vi "Start test 1.vi"(8 "error in (no error)":errorcluster, 11 "Test_ExampleClassA in":refnum<class "Test_ExampleClassA.lvclass">) -> (0 "error out":errorcluster, 3 "Test_ExampleClassA out":refnum<class "Test_ExampleClassA.lvclass">)   [LabVIEW 2012, in "Test_ExampleClassA.lvclass"]
doc: "Starts test 1 (i.e. the second default test). Sends an update command together with a complete set of settings to test whether an acknowledge command is returned."
uses:
  Test_ExampleClassA.lvclass
  Test settings cluster.ctl
  ExampleClassA/Settings cluster.ctl
  MurmexTest/MurmexTest.lvclass
  ExampleClassA/ExampleClassA.lvclass
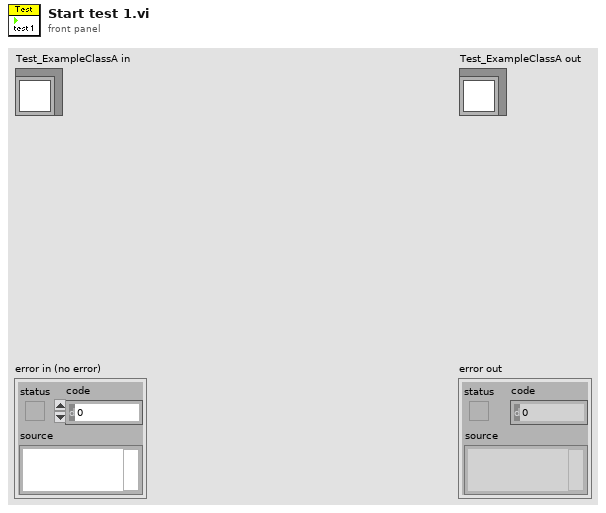
[diagram p1: front panel]
types:
  T1 = typedef "Test_ExampleClassA.lvclass/Test settings cluster.ctl" = cluster{"settings":T2, "valid?":bool}
  T2 = typedef "ExampleClassA.lvclass/Settings cluster.ctl" = cluster{"period?":dbl[unit], "number of blocks":i32, "number of channels":i32}
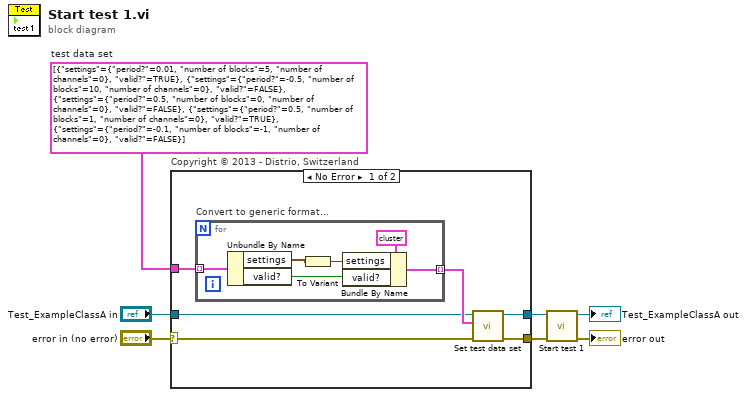
[diagram p0: block diagram]
diagram:
  w1 = T1[] [{"settings"={"period?"=0.01, "number of blocks"=5, "number of channels"=0}, "valid?"=TRUE}, {"settings"={"period?"=-0.5, "number of blocks"=10, "number of channels"=0}, "valid?"=FALSE}, {"settings"={"period?"=0.5, "number of blocks"=0, "number of channels"=0}, "valid?"=FALSE}, {"settings"={"period?"=0.5, "number of blocks"=1, "number of channels"=0}, "valid?"=TRUE}, {"settings"={"period?"=-0.1, "number of blocks"=-1, "number of channels"=0}, "valid?"=FALSE}]  # test data set
  n1 = case "Copyright © 2013 - Distrio, Switzerland" shown="No Error" "error in (no error)" {
    selector: "error in (no error)" -> [w9 w21]
    tunnel: "Test_ExampleClassA in" -> [w11 w20]
    tunnel: [w8 w21] -> w3
    tunnel: [w10 w20] -> w2
    tunnel: w1 -> [w13 _]
    frame No Error {
      n2 = for "Convert to generic format..." {
        tunnel: w13 -> [w19] mode=indexing
        tunnel: [w14] -> w12 mode=indexing
        n3 = Unbundle By Name(w19) -> ("settings"=w15:T2, "valid?"=w17:bool)
        n4 = To Variant(anything=w15) -> (Variant=w16:variant)
        n5 = Bundle By Name(cluster=cluster{"settings":variant, "valid?":bool} {"settings"=variant, "valid?"=FALSE} ("test settings"), "settings"=w16, "valid?"=w17) -> (w14:cluster{"settings":variant, "valid?":bool})
      }
      n6 = call "Set test data set.vi"("error in (no error)"=w9, "test settings"=w12, "MurmexTest in"=w11) -> ("error out"=w8:errorcluster, "MurmexTest out"=w10:refnum<class "Test_ExampleClassA.lvclass">)  [unwired: 7 in]
    }
    frame Error {
    }
  }
  n7 = call-parent "Start test 1.vi"("error in (no error)"=w3, "MurmexTest in"=w2) -> ("error out"=→"error out":errorcluster, "MurmexTest out"=→"Test_ExampleClassA out":refnum<class "Test_ExampleClassA.lvclass">)  [unwired: 8 in]
